vi "FTW-Test-CSV-Array.vi"() -> ()   [LabVIEW 2015]
panel:
  out "CSV String":string
  out "error out":errorcluster
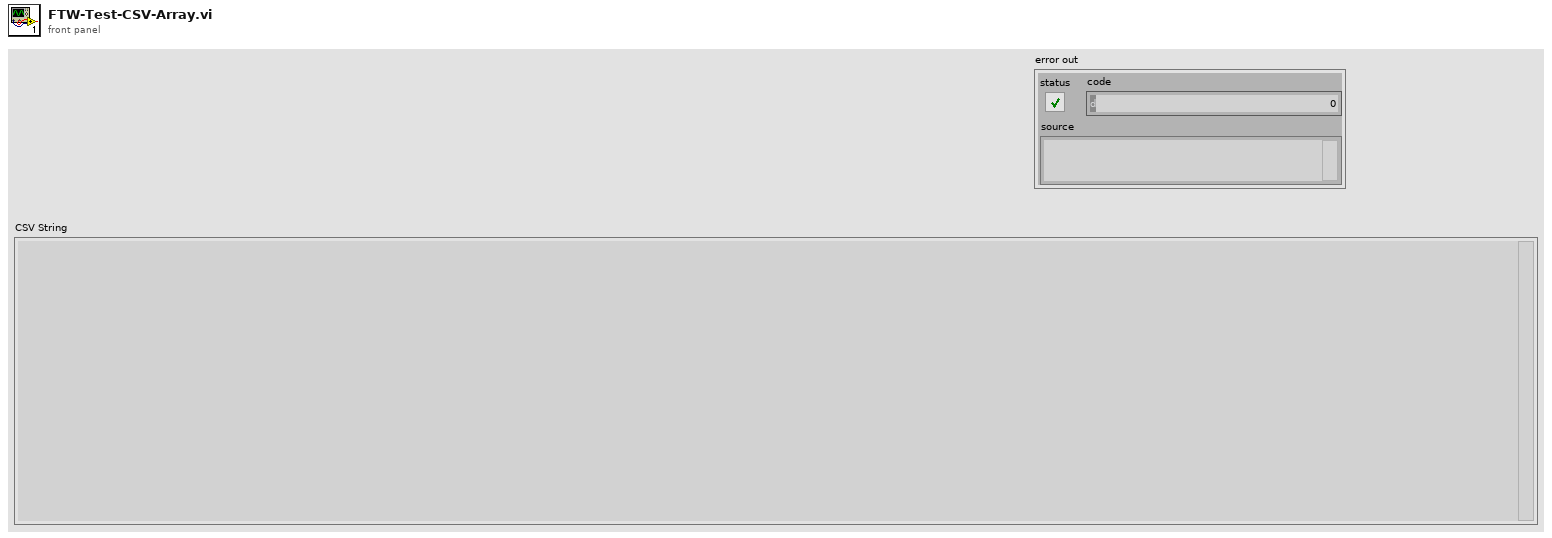
[diagram p1: front panel]
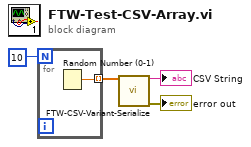
[diagram p0: block diagram]
diagram:
  n1 = for {
    N: 10 -> [_]
    tunnel: [w5] -> w1 mode=indexing
    n2 = Random Number (0-1)() -> (number: 0 to 1=w5:dbl)
  }
  n3 = call "FTW-CSV-Variant-Serialize.vi"("Variant"=w1) -> ("CSV String"=→"CSV String":string, "error out"=→"error out":errorcluster)  [unwired: 13 in]
